vi "Zero Phase Filter (DBL).vi"(9 "Forward Coefficients":dbl[](array[numeric]), 10 "Reverse Coefficients":dbl[](array[numeric]), 11 "X":dbl[](array[numeric])) -> (0 "error":i32, 3 "Filtered X":dbl[](array[numeric]))   [LabVIEW 2017, in "NI_AALBase.lvlib"]
doc: "Applies a zero phase filter to an input sequence <B>X</B>. Wire data to the <B>X</B> input to determine the polymorphic instance to use or manually select the instance."
uses:
  NI_AALBase.lvlib
  lvanlys.dll
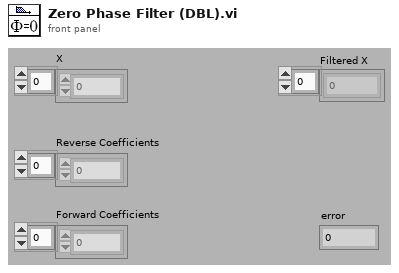
[diagram p1: front panel]
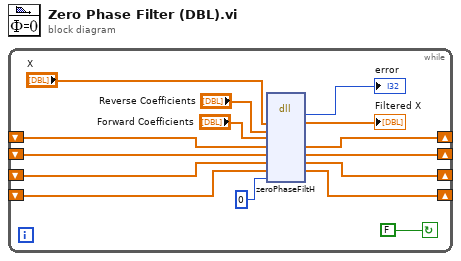
[diagram p0: block diagram]
diagram:
  n1 = while {
    shift-left: _ -> [w8]
    shift-right: [w9] -> _
    shift-left: _ -> [w10]
    shift-right: [w11] -> _
    shift-right: [w7] -> _
    shift-left: _ -> [w6]
    shift-right: [w5] -> _
    shift-left: _ -> [w4]
    stop <- FALSE continue-if-true
    n2 = dll-call lib="C:/Program Files/National Instruments/LabVIEW 2017/resource/lvanlys.*" fn="zeroPhaseFiltH"("X"="X", "Reverse Coefficients"="Reverse Coefficients", "Forward Coefficients"="Forward Coefficients", "x1H"=w10, "x2H"=w8, "y1H"=w6, "y2H"=w4, "reset"=0) -> (→"error":i32, "X"=→"Filtered X":dbl[], "x1H"=w11:dbl[], "x2H"=w9:dbl[], "y1H"=w7:dbl[], "y2H"=w5:dbl[])  [unwired: 6 in, 2 out]
  }
